vi "SWITCH Action-Status.vi"(8 "error in (no error)":errorcluster, 10 "Message Data":variant, 11 "Data Cluster":T1={"Tango HW"={"VISA resource"="", "Baud Rate (115200)"=2, "lAnInterfaceType"=0, "bAShowProt"=15}, "Writer Queue"=refnum, "Status"=FALSE, "Abs Position"=[], "Axis Velocity"={"dX"=0.0, "dY"=0.0, "dZ"=0.0, "dA"=0.0}, "acceleration "=0.0, "Z direction"=enum."Up", "Position Mode"="", "plLSID"=0}) -> (0 "error out":errorcluster, 3 "Data Cluster out":T1={"Tango HW"={"VISA resource"="", "Baud Rate (115200)"=2, "lAnInterfaceType"=0, "bAShowProt"=15}, "Writer Queue"=refnum, "Status"=FALSE, "Abs Position"=[], "Axis Velocity"={"dX"=0.0, "dY"=0.0, "dZ"=0.0, "dA"=0.0}, "acceleration "=0.0, "Z direction"=enum."Up", "Position Mode"="", "plLSID"=0})   [LabVIEW 2020, in "MOTOR.lvlib"]
uses:
  MOTOR.lvlib
  PS Hardware Configuration.ctl
  support/Message Queue/Message Cluster.ctl
  support/Message Queue/Message Queue.lvlib
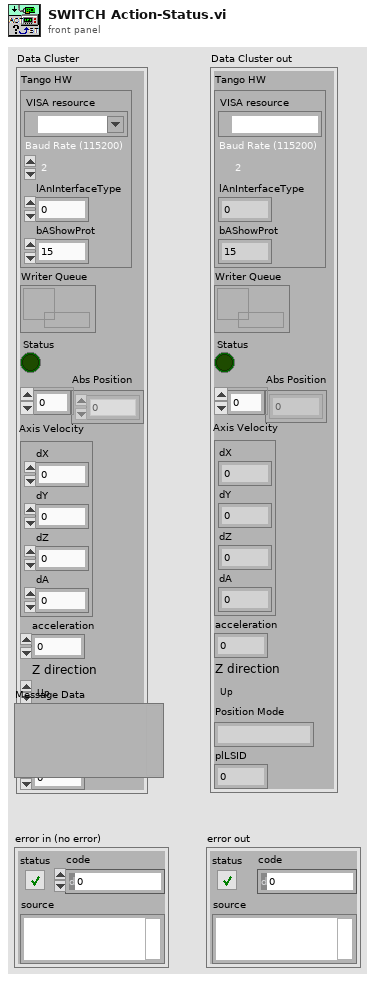
[diagram p1: front panel]
types:
  T1 = typedef "MOTOR.lvlib/PS Hardware Configuration.ctl" = cluster{"Tango HW":cluster{"VISA resource":refnum<visa-resource-name>, "Baud Rate (115200)":i32, "lAnInterfaceType":i32, "bAShowProt":i32}, "Writer Queue":refnum<queue>, "Status":bool, "Abs Position":i32[], "Axis Velocity":cluster{"dX":dbl, "dY":dbl, "dZ":dbl, "dA":dbl}, "acceleration ":dbl, "Z direction":enum16{"Up", "Down"}, "Position Mode":string, "plLSID":i32}
  T2 = typedef "Message Queue.lvlib/Message Cluster.ctl" = cluster{"Message":string, "Message Data":variant}
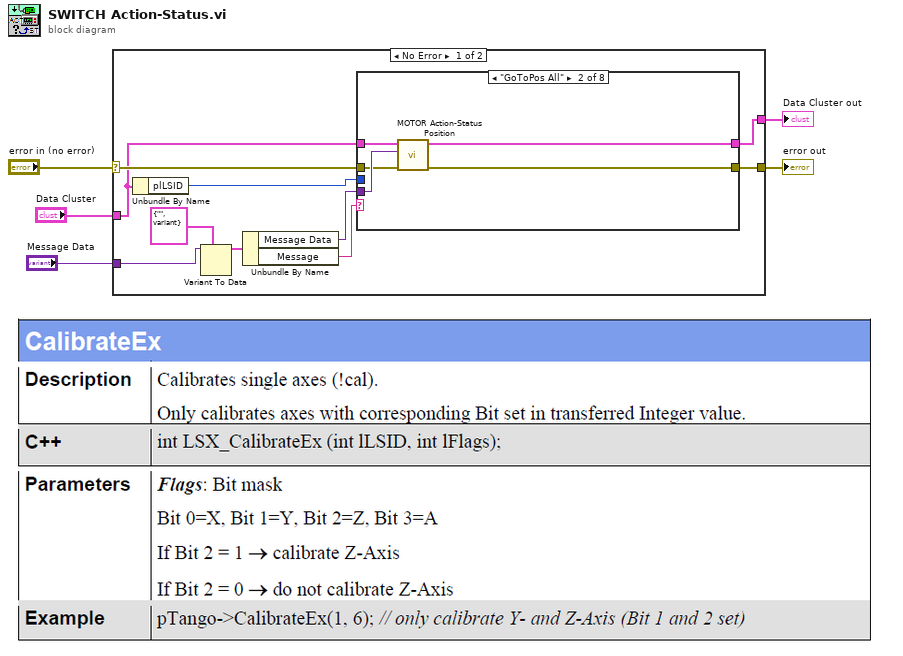
[diagram p0: block diagram]
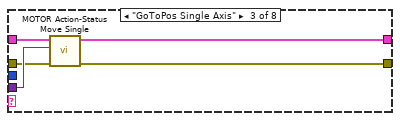
[diagram p3: hidden frame]
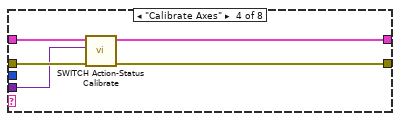
[diagram p4: hidden frame]
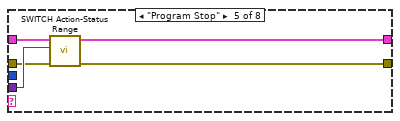
[diagram p5: hidden frame]
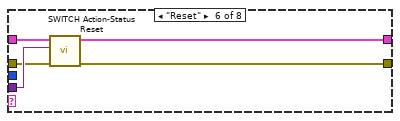
[diagram p6: hidden frame]
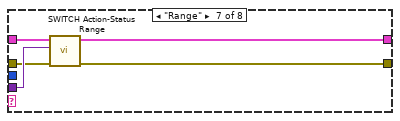
[diagram p7: hidden frame]
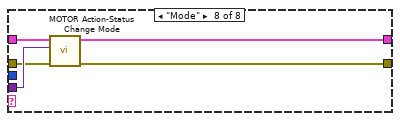
[diagram p8: hidden frame]
diagram:
  n1 = case shown="No Error" "error in (no error)" {
    selector: "error in (no error)" -> [w9 w53]
    tunnel: [w15 w53] -> w5
    tunnel: "Data Cluster" -> [w7 w54]
    tunnel: [w14 w54] -> w3
    tunnel: "Message Data" -> [w10 _]
    frame No Error {
      n2 = Unbundle By Name(w7) -> ("plLSID"=w6:i32)
      n3 = Variant To Data(type=T2 {"Message"="", "Message Data"=variant} ("element"), Variant=w10) -> (data=w12:T2)  [unwired: 1 in, 1 out]
      n4 = Unbundle By Name(w12) -> ("Message Data"=w8:variant, "Message"=w13:string)
      n5 = case shown="\"GoToPos All\"" w13 {
        tunnel: w8 -> [_ w21 w26 w31 w36 w41 w46 w50]
        tunnel: [w17 w20 w24 w29 w35 w40 w45 w51] -> w14
        tunnel: w7 -> [w17 w22 w27 w30 w37 w42 w47 w52]
        tunnel: w9 -> [w16 w18 w25 w32 w33 w38 w43 w49]
        tunnel: [w16 w19 w23 w28 w34 w39 w44 w48] -> w15
        tunnel: w6 -> [_ _ _ _ _ _ _ _]
        frame "False", Default {
        }
        frame "GoToPos All" {
          n6 = call "MOTOR Action-Status Position.vi"("error in (no error)"=w18, "Message Data"=w21, "Data Cluster in"=w22) -> ("error out"=w19:errorcluster, "Data Cluster out"=w20:T1)  [unwired: 7 in]
        }
        frame "GoToPos Single Axis" {
          n7 = call "MOTOR Action-Status Move Single.vi"("error in (no error)"=w25, "Message Data"=w26, "Data Cluster in"=w27) -> ("error out"=w23:errorcluster, "Data Cluster out"=w24:T1)  [unwired: 7 in]
        }
        frame "Calibrate Axes" {
          n8 = call "SWITCH Action-Status Calibrate.vi"("error in (no error)"=w32, "Message Data"=w31, "Data Cluster in"=w30) -> ("error out"=w28:errorcluster, "Data Cluster out"=w29:T1)  [unwired: 7 in]
        }
        frame "Program Stop" {
          n9 = call "SWITCH Action-Status Range.vi"("error in (no error)"=w33, "Message Data"=w36, "Data Cluster in"=w37) -> ("error out"=w34:errorcluster, "Data Cluster out"=w35:T1)  [unwired: 7 in]
        }
        frame "Reset" {
          n10 = call "SWITCH Action-Status Reset.vi"("error in (no error)"=w38, "Message Data"=w41, "Data Cluster in"=w42) -> ("error out"=w39:errorcluster, "Data Cluster out"=w40:T1)  [unwired: 7 in]
        }
        frame "Range" {
          n11 = call "SWITCH Action-Status Range.vi"("error in (no error)"=w43, "Message Data"=w46, "Data Cluster in"=w47) -> ("error out"=w44:errorcluster, "Data Cluster out"=w45:T1)  [unwired: 7 in]
        }
        frame "Mode" {
          n12 = call "MOTOR Action-Status Change Mode.vi"("error in (no error)"=w49, "Message Data"=w50, "Data Cluster in"=w52) -> ("error out"=w48:errorcluster, "Data Cluster out"=w51:T1)  [unwired: 7 in]
        }
      }
    }
    frame Error {
    }
  }
  "error out" <- w5
  "Data Cluster out" <- w3
